vi "Thermo Instrument UI.vi"() -> ()   [LabVIEW 2025, in "Thermo.lvlib" / "Thermo Instrument.lvclass"]
doc: "Copyright 2017 National Instruments Corporation\n\nLicensed under the Apache License, Version 2.0 (the \"License\"); you may not use this file except in compliance with the License. You may obtain a copy of the License at http://www.apache.org/licenses/LICENSE-2.0\nUnless required by applicable law or agreed to in writing, software distributed under the License is distributed on an \"AS IS\" BASIS, WITHOUT WARRANTIES OR CONDITIONS OF ANY KIND, either express or implied. See the License for the specific language governing permissions and limitations under the License."
uses:
  Thermo Instrument.lvclass
  Thermo Instrument.lvclass/Thermo Instrument.ctl
  Users/Public/Documents/Sandia National Labs/TSS Plugin/CEF.lvlibp/Node/CEF_Node.lvclass
  Thermo configuration/Thermo configuration.lvclass
  Users/Public/Documents/Sandia National Labs/TSS Plugin/CEF.lvlibp/Node/NodeRef.ctl
  Users/Public/Documents/Sandia National Labs/TSS Plugin/CEF.lvlibp/Node/UserEventRef.ctl
  Users/Public/Documents/Sandia National Labs/TSS Plugin/CEF.lvlibp/Node/mainQref.ctl
  Thermo configuration/Thermo Setting.ctl
  Users/Public/Documents/Sandia National Labs/TSS Plugin/Abstract Engine.lvlibp/Instrument configuration/Default Instrument.ctl
  Users/Public/Documents/Sandia National Labs/TSS Plugin/Abstract Engine.lvlibp/Instrument configuration/Instrument configuration.lvclass
panel:
  in  "Instrument":cluster{"Default":T1, "Setting":T2}={"Default"={"Type"="None", "Address"="localhost", "SW Alias"="", "Description"="* Type = Node Class", "Enabled"=TRUE}, "Setting"={"Numeric"=0.5, "Combo"="", "String"="", "Boolean"=FALSE}} {"Setting"."Numeric" format="%#_f"}
  in  "user event":T3
  in  "main queue":T4
  in  "node ref":T5
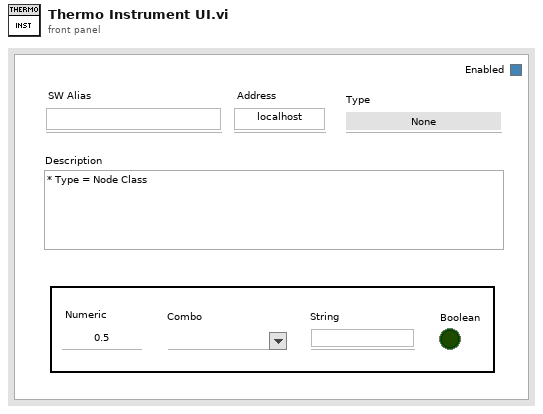
[diagram p1: front panel]
types:
  T1 = typedef "Abstract Engine.lvlibp/Instrument configuration.lvclass/Default Instrument.ctl" = cluster{"Type":string, "Address":string, "SW Alias":string, "Description":string, "Enabled":bool}
  T2 = typedef "Thermo.lvlib/Thermo configuration.lvclass/Thermo Setting.ctl" = cluster{"Numeric":dbl, "Combo":string, "String":string, "Boolean":bool}
  T3 = typedef "CEF.lvlibp/CEF_Node.lvclass/UserEventRef.ctl" = refnum<user-event>
  T4 = typedef "CEF.lvlibp/CEF_Node.lvclass/mainQref.ctl" = refnum<queue>
  T5 = typedef "CEF.lvlibp/CEF_Node.lvclass/NodeRef.ctl" = refnum<data-value>
  T6 = cluster{"Instrument Setting":T1, "Thermo Setting":T2}
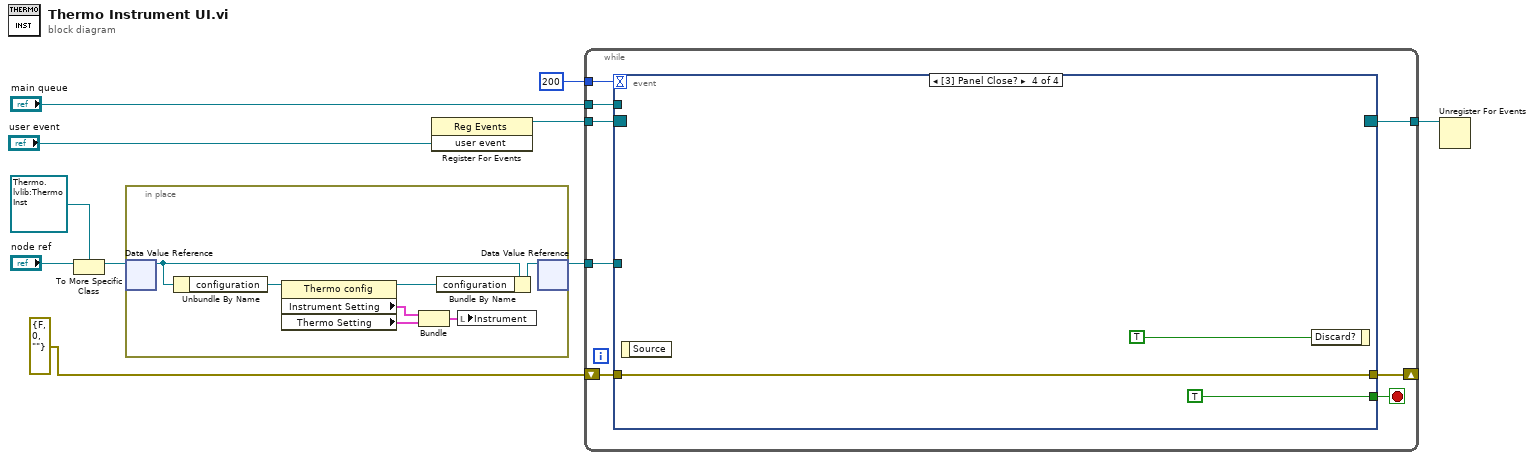
[diagram p0: block diagram]
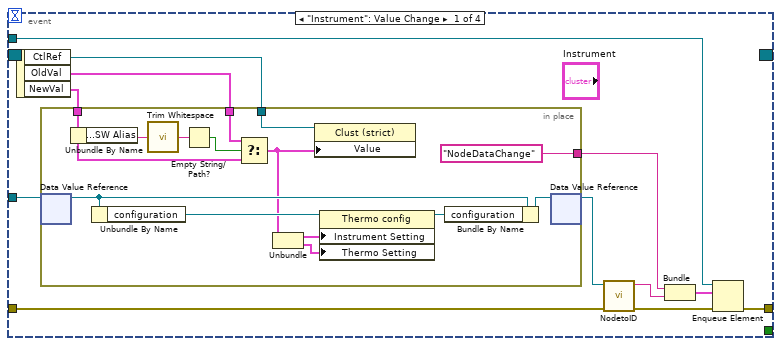
[diagram p2: hidden frame]
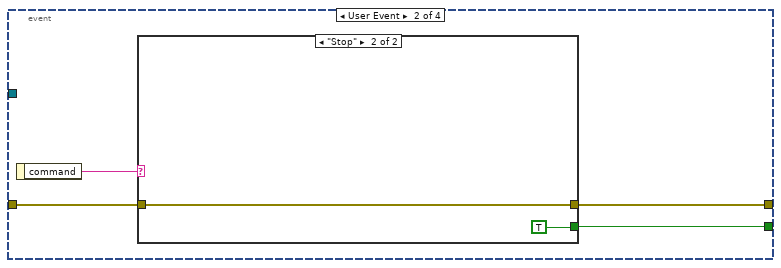
[diagram p3: hidden frame]
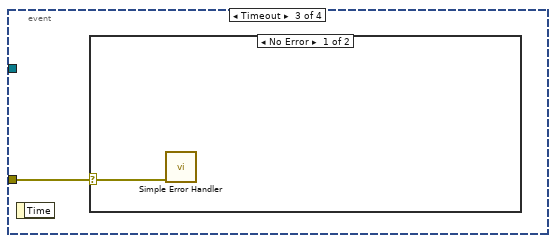
[diagram p5: hidden frame]
diagram:
  n1 = To More Specific Class(target class=refnum<data-value> refnum ("data value reference"), reference="node ref") -> (specific class reference=w6:refnum<data-value>)  [unwired: 1 in, 1 out]
  n2 = in-place {
    # "Initialize the front panel controls when loaded"
    n3 = in-place-dvr #1(w6) -> (w17:refnum<class "Thermo Instrument.lvclass">)  [unwired: 1 out]
    n4 = Unbundle By Name(w17) -> ("configuration"=w16:refnum<class "Thermo configuration.lvclass">)
    n5 = property class="Thermo config"(reference=w16) -> (reference out=w14:refnum<class "Thermo configuration.lvclass">, "Instrument Setting"=w12:T1, "Thermo Setting"=w11:T2)  [unwired: 1 in, 1 out]
    n6 = Bundle("Instrument Setting"=w12, "Thermo Setting"=w11) -> (w13:T6)  [unwired: 1 in]
    n7 = Bundle By Name(cluster=w17, "configuration"=w14) -> (w15:refnum<class "Thermo Instrument.lvclass">)
    n8 = local write "Instrument"(w13) -> ()
    n9 = in-place-dvr #1(w15) -> (w5:refnum<data-value>)  [unwired: 1 out]
  }
  n10 = register-events("user event") -> (reference out=w9:refnum<event-registration>)  [unwired: 2 in, 1 out]
  n11 = while {
    tunnel: w5 -> [w25]
    tunnel: w9 -> [w24]
    tunnel: [w23] -> w8
    tunnel: "main queue" -> [w19]
    tunnel: 200 -> [w18]
    shift-right: [w20] -> _
    shift-left: errorcluster {"status"=FALSE, "code"=0, "source"=""} ("error out") -> [w21]
    stop <- w22 stop-if-true
    n12 = event shown="[3] Panel Close?" {
      selector: w24 -> [_ _ _ _]
      dyn-events: [_ _ _ _] -> w23
      timeout: w18 -> [_ _ _ _]
      tunnel: w25 -> [w37 _ _ _]
      tunnel: [_ w55 _ TRUE] -> w22
      tunnel: [w32 w52 _ w61] -> w20
      tunnel: w21 -> [w27 w54 w59 w61]
      tunnel: w19 -> [w31 _ _ _]
      event "Instrument": Value Change {
        n13 = event-data() -> ("CtlRef"=w34:refnum<vi>, "OldVal"=w35:cluster{"Default":T1, "Setting":T2}, "NewVal"=w36:cluster{"Default":T1, "Setting":T2})  [unwired: 1 in]
        n14 = in-place {
          in-place-border: w35 -> [w48]
          in-place-border: w34 -> [w47]
          in-place-border: w36 -> [w41]
          in-place-border: ["NodeDataChange" ("Message Name")] -> w30
          n15 = in-place-dvr #2(w37) -> (w51:refnum<class "Thermo Instrument.lvclass">)  [unwired: 1 out]
          n16 = Unbundle By Name(w41) -> ("Default.SW Alias"=w40:string)
          n17 = Unbundle By Name(w51) -> ("configuration"=w46:refnum<class "Thermo configuration.lvclass">)
          n18 = call <vilib>:"Trim Whitespace.vi"("string"=w40) -> ("trimmed string"=w43:string)  [unwired: 1 in]
          n19 = Empty String/Path?(string/path=w43) -> (empty?=w42:bool)
          n20 = Select(t=w48, s=w42, f=w41) -> (s? t:f=w45:cluster{"Default":T1, "Setting":T2})
          n21 = Unbundle(w45) -> ("Default"=w44:T1, "Setting"=w39:T2)
          n22 = property class="Clust (strict)"(reference=w47, "Value"=w45) -> ()  [unwired: 1 in, 2 out]
          n23 = property class="Thermo config"(reference=w46, "Instrument Setting"=w44, "Thermo Setting"=w39) -> (reference out=w50:refnum<class "Thermo configuration.lvclass">)  [unwired: 1 in, 1 out]
          n24 = Bundle By Name(cluster=w51, "configuration"=w50) -> (w49:refnum<class "Thermo Instrument.lvclass">)
          n25 = in-place-dvr #2(w49) -> (w33:refnum<data-value>)  [unwired: 1 out]
        }
        n26 = call "NodetoID.vi"("error in"=w27, "node ref"=w33) -> ("error out"=w26:errorcluster, "ID"=w29:string)  [unwired: 8 in]
        n27 = Bundle("Message Name"=w30, "ID"=w29) -> (w28:cluster{"Message Name":string, "ID":string})  [unwired: 1 in]
        n28 = Enqueue Element(queue=w31, element=w28, error in (no error)=w26) -> (error out=w32:errorcluster)  [unwired: 1 in, 2 out]
      }
      event User Event {
        n29 = event-data() -> ("command"=w53:string)  [unwired: 1 in]
        n30 = case shown="\"Stop\"" w53 {
          tunnel: [_ TRUE] -> w55
          tunnel: w54 -> [w56 w57]
          tunnel: [w56 w57] -> w52
          frame Default {
          }
          frame "Stop" {
          }
        }
      }
      event Timeout {
        n31 = event-data() -> ()  [unwired: 1 in, 1 out]
        n32 = case shown="No Error" w59 {
          selector: w59 -> [w60 _]
          frame No Error {
            n33 = call <vilib>:"Simple Error Handler.vi"("error in (no error)"=w60) -> ()  [unwired: 4 in, 5 out]
          }
          frame Error {
          }
        }
      }
      event Panel Close? {
        n34 = event-data() -> ()  [unwired: 1 in, 1 out]
        n35 = event-data("Discard?"=TRUE) -> ()  [unwired: 1 in, 1 out]
      }
    }
  }
  n36 = Unregister For Events(event registration refnum=w8) -> ()  [unwired: 1 in, 1 out]
